vi "EHL Filter - Value Change MHLC.vi"(8 "error in (no error)":errorcluster, 11 "Message Log in":refnum<class "Message Log.lvclass">) -> (0 "error out":errorcluster, 3 "Message Log out":refnum<class "Message Log.lvclass">)   [LabVIEW 2017, in "Message Log.lvclass"]
doc: "Filter Button has been pressed. Add Element to Filter Data and update the Message Log with the filtered data"
uses:
  Message Log.lvclass
  Message Log.lvclass/Message Log.ctl
  <vilib>/Utility/miscctls.llb/LVRowAndColumnUnsignedTypeDef.ctl
  Message Log Filter Data.ctl
  Message Log Columns.ctl
  String Filter Type.ctl
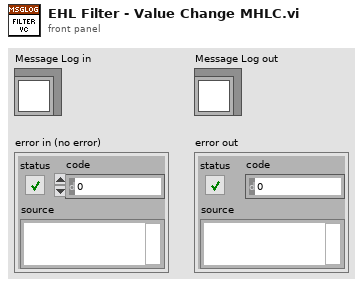
[diagram p1: front panel]
types:
  T1 = typedef "Debug Server OLD.lvclass/Message Log Columns.ctl" = enum16{"Count (sec)", "Time/Date", "Enque Worker", "Enque Case", "Deque Worker", "Deque Case", "Priority", "Message"}
  T2 = typedef "Message Log.lvclass/Message Log Filter Data.ctl" = cluster{"Element":string, "Column":T3, "Filter Type":T4}
  T3 = typedef "Message Log.lvclass/Message Log Columns.ctl" = enum16{"Count (sec)", "Time/Date", "Enque Worker", "Enque Case", "Deque Worker", "Deque Case", "Priority", "Message"}
  T4 = typedef "Message Log.lvclass/String Filter Type.ctl" = enum16{"string only", "match pattern"}
  T5 = typedef "LVRowAndColumnUnsignedTypeDef.ctl" = cluster{"Row":u32, "Column":u32}
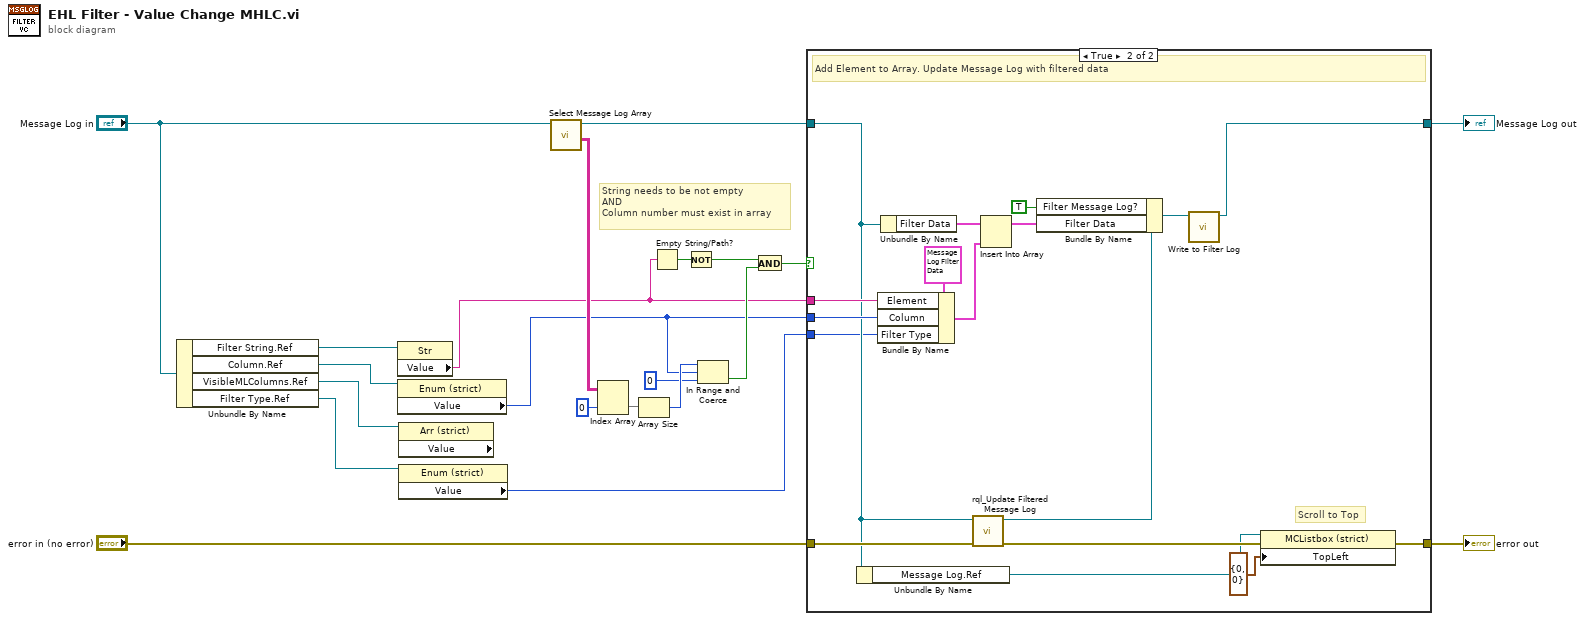
[diagram p0: block diagram]
diagram:
  # "String needs to be not empty\nAND\nColumn number must exist in array"
  n1 = Unbundle By Name("Message Log in") -> ("Filter String.Ref"=w7:refnum<vi>, "Column.Ref"=w6:refnum<vi>, "VisibleMLColumns.Ref"=w4:refnum<vi>, "Filter Type.Ref"=w3:refnum<vi>)
  n2 = property class="Str"(reference=w7) -> ("Value"=w5:string)  [unwired: 1 in, 2 out]
  n3 = property class="Enum (strict)"(reference=w6) -> ("Value"=w1:T1)  [unwired: 1 in, 2 out]
  n4 = property class="Arr (strict)" props=["Value"](reference=w4) -> ()  [unwired: 1 in, 3 out]
  n5 = property class="Enum (strict)"(reference=w3) -> ("Value"=w2:enum16{"string only", "match pattern"})  [unwired: 1 in, 2 out]
  n6 = call "Select Message Log Array.vi"("Message Log in"="Message Log in") -> ("Selected Array"=w20:string[][], "Message Log out"=w21:refnum<class "Message Log.lvclass">)  [unwired: 9 in]
  n7 = Index Array(array=w20, index (row)=0) -> (element=w13:string[])  [unwired: 1 in]
  n8 = Array Size(array=w13) -> (size(s)=w18:i32)
  n9 = Empty String/Path?(string/path=w5) -> (empty?=w14:bool)
  n10 = Not(x=w14) -> (.not. x?=w19:bool)
  n11 = In Range and Coerce(upper limit=w18, x=w1, lower limit=0) -> (In Range?=w16:bool)  [unwired: 1 out]
  n12 = And(x=w19, y=w16) -> (x .and. y?=w15:bool)
  n13 = case shown="True" w15 {
    tunnel: [w23 w37] -> w9
    tunnel: "error in (no error)" -> [w23 w39]
    tunnel: w21 -> [w22 w28]
    tunnel: [w22 w25] -> w10
    tunnel: w5 -> [_ w31]
    tunnel: w1 -> [_ w30]
    tunnel: w2 -> [_ w24]
    frame False {
      # "Unsuccessful setting up filter parameters. Do Nothing"
    }
    frame True {
      # "Scroll to Top"
      # "Add Element to Array. Update Message Log with filtered data"
      n14 = Unbundle By Name(w28) -> ("Message Log.Ref"=w36:refnum<vi>)
      n15 = Bundle By Name(cluster=T2 {"Element"="", "Column"=enum."Count (sec)", "Filter Type"=enum."string only"} ("Message Log Filter Data"), "Element"=w31, "Column"=w30, "Filter Type"=w24) -> (w33:T2)
      n16 = Unbundle By Name(w28) -> ("Filter Data"=w34:T2[])
      n17 = call "rql_Update Filtered Message Log.vi"("error in"=w39, "Message Log in"=w28) -> ("error out"=w38:errorcluster, "dup Message Log out"=w27:refnum<class "Message Log.lvclass">)  [unwired: 8 in]
      n18 = Insert Into Array(array=w34, new element=w33) -> (w35:T2[])  [unwired: 1 in]
      n19 = Bundle By Name(cluster=w27, "Filter Message Log?"=TRUE, "Filter Data"=w35) -> (w26:refnum<class "Message Log.lvclass">)
      n20 = call "Write to Filter Log.vi"("Message Log in"=w26) -> ("Message Log out"=w25:refnum<class "Message Log.lvclass">)  [unwired: 9 in, 1 out]
      n21 = property class="MCListbox (strict)"(reference=w36, error in=w38, "TopLeft"=T5 {"Row"=0, "Column"=0} ("Top Left Visible Cell")) -> (error out=w37:errorcluster)  [unwired: 1 out]
    }
  }
  "Message Log out" <- w10
  "error out" <- w9
